vi "ramp.vi"(0 "input":sgl, 1 "rampRate":sgl, 11 "stateIn":sgl format="%#_13g", 12 "Resources":T1) -> (4 "output":sgl)   [LabVIEW 2017]
uses:
  Adder/Adder.lvclass
  Subtractor/Subtractor.lvclass
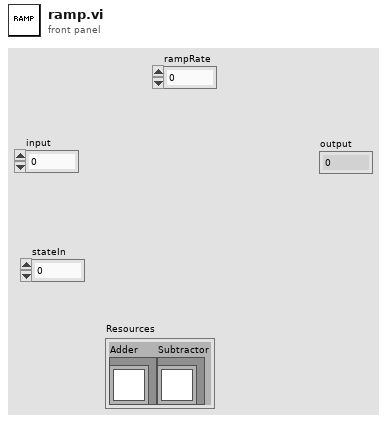
[diagram p1: front panel]
types:
  T1 = cluster{"Adder":refnum<class "Adder.lvclass">, "Subtractor":refnum<class "Subtractor.lvclass">}
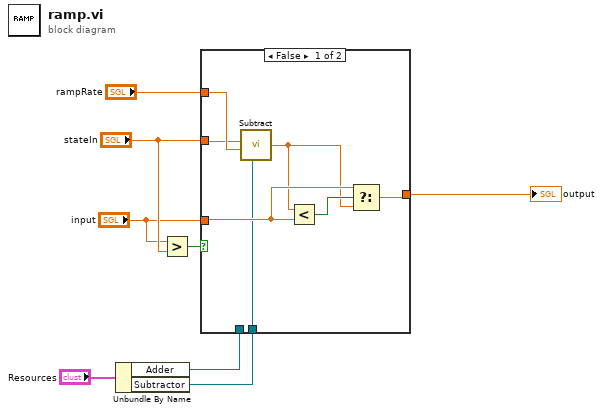
[diagram p0: block diagram]
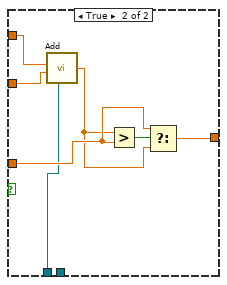
[diagram p2: hidden frame]
diagram:
  n1 = Unbundle By Name("Resources") -> ("Adder"=w1:refnum<class "Adder.lvclass">, "Subtractor"=w2:refnum<class "Subtractor.lvclass">)
  n2 = Greater?(x="input", y="stateIn") -> (0:w5:bool)
  n3 = case shown="False" w5 {
    tunnel: "rampRate" -> [w12 w19]
    tunnel: "stateIn" -> [w10 w18]
    tunnel: "input" -> [w13 w20]
    tunnel: [w14 w21] -> w4
    tunnel: w2 -> [w9 _]
    tunnel: w1 -> [_ w16]
    frame False {
      n4 = call-dynamic "Subtract.vi"("x"=w10, "y"=w12, "Subtractor"=w9) -> ("x-y"=w11:sgl)  [unwired: 4 in]
      n5 = Less?(x=w11, y=w13) -> (x < y?=w15:bool)
      n6 = Select(t=w13, s=w15, f=w11) -> (s? t:f=w14:sgl)
    }
    frame True {
      n7 = call-dynamic "Add.vi"("x"=w19, "y"=w18, "Adder"=w16) -> ("x+y"=w17:sgl)  [unwired: 4 in]
      n8 = Greater?(x=w17, y=w20) -> (0:w22:bool)
      n9 = Select(t=w20, s=w22, f=w17) -> (s? t:f=w21:sgl)
    }
  }
  "output" <- w4
